vi "RT Driver VI.vi"(6 "Device Clock":string, 9 "Device Inputs FIFO":refnum<k33>, 10 "Device Outputs FIFO":refnum<k33>, 11 "Device Reference":T1 format="%.0x") -> ()   [LabVIEW 2016, in "UDP CD Engine.lvlib"]
uses:
  <vilib>/NI Veristand/Custom Device API/Custom Device Item Ref.ctl
  <vilib>/NI Veristand/Custom Device API/Custom Device Channel Type.ctl
  <vilib>/NI Veristand/Custom Device API/Message Response (String).ctl
  <vilib>/NI Veristand/Custom Device API/Message Response (Byte Array).ctl
  UDP CD Engine.lvlib
  <vilib>/NI Veristand/Custom Device API/Custom Device API.lvlib
  <vilib>/NI Veristand/Custom Device Tools/Custom Device Utility Library/Custom Device Utility Library.lvlib
panel:
  in  "Initialization Status Notifier":refnum<notifier>
  in  "Status Notifier":refnum<notifier>
  # "Custom Device Template\nv1.0"
  # "Use this template as a starting point for creating a custom device code module. The input controls shown here are specially named controls that the system will use to provide the device loop with data. The controls are not required for the device loop to run. For instance, if the device doesn't produce any output data, then you don't need the Device Outputs FIFO control. If you do use these controls, however, they need to have these exact names to be functional."
  # "The optional status notifier element is used to notify the RT engine of the last state of the custom device, and to indicate the device has completed execution. If this control is not used, a default No Error value is returned to the system when the device finishes execution.\n\nNote: This error state is not checked until the system shuts down. Use an output status channel to send more immediate status values to the system."
  # "This optional input can be used to send the VeriStand Engine the final status of the custom device initalization process. If this control exists on the custom device front panel, the VeriStand Engine will wait for a status update before starting up. If the custom device reports an error, that will abort the execution of the current configuration in the VeriStand Engine.\n\nThis control can be deleted if the custom device does not need to send the initialization status update."
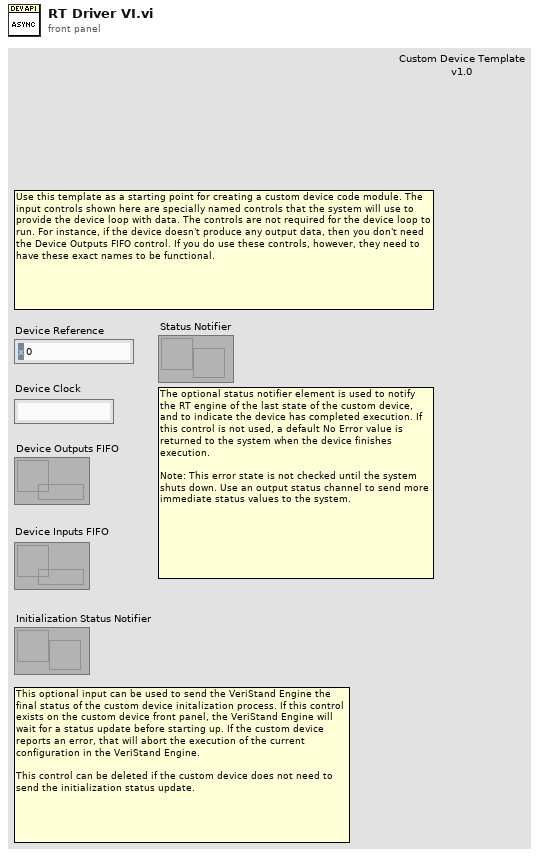
[diagram p1: front panel]
types:
  T1 = typedef "Custom Device API.lvlib/Custom Device Item Ref.ctl" = u64
  T2 = typedef "Custom Device API.lvlib/Custom Device Channel Type.ctl" = enum16{"Input", "Output"}
  T3 = typedef "Custom Device API.lvlib/Custom Device Engine Event Ref.ctl" = refnum<event-registration>
  T4 = typedef "Custom Device API.lvlib/Message Response (String).ctl" = cluster{"Response":string, "Error":errorcluster}
  T5 = typedef "Custom Device API.lvlib/Message Response (Byte Array).ctl" = cluster{"Response":u8[], "Error":errorcluster}
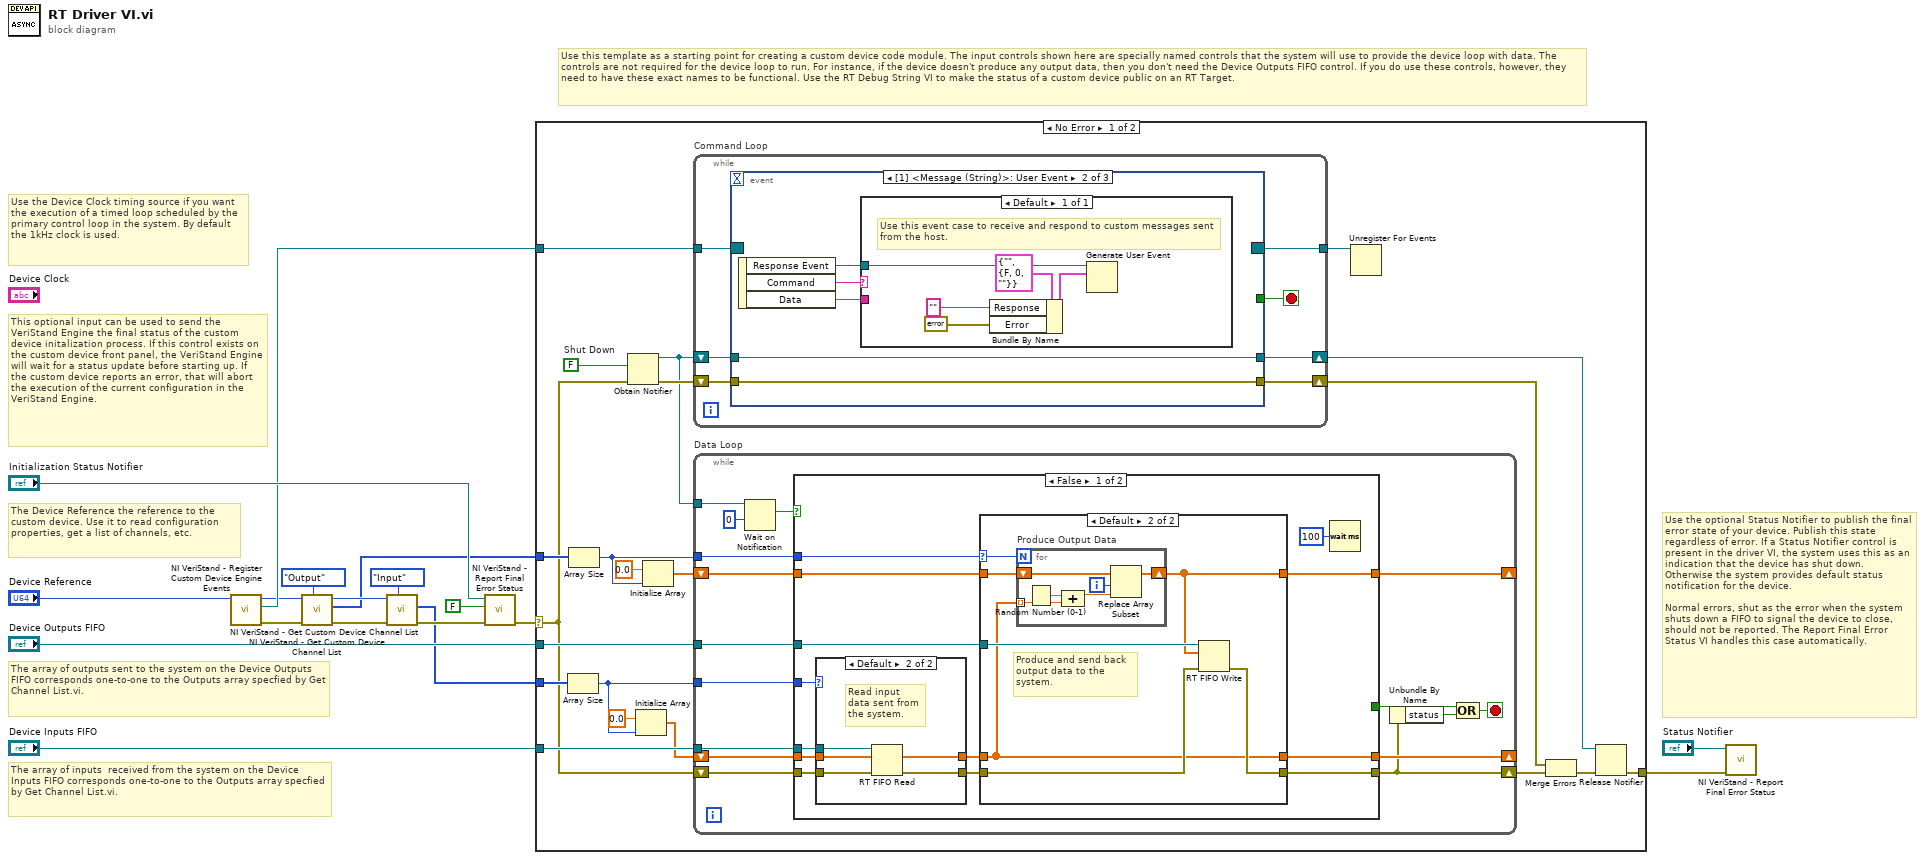
[diagram p0: block diagram]
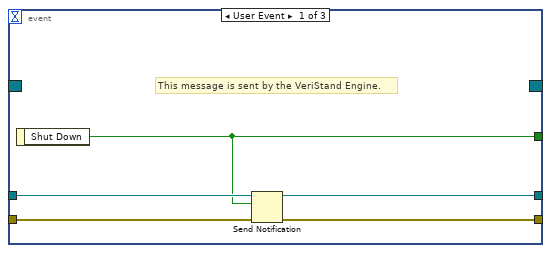
[diagram p2: hidden frame]
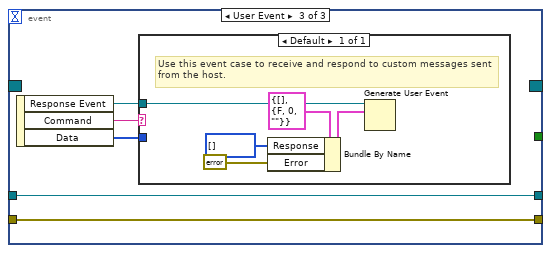
[diagram p3: hidden frame]
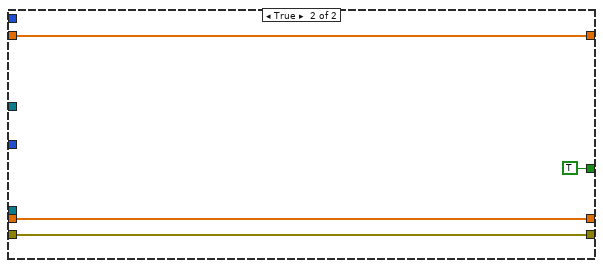
[diagram p6: hidden frame]
diagram:
  # "This optional input can be used to send the VeriStand Engine the final status of the custom device initalization process. If this control exists on the custom device front panel, the VeriStand Engine will wait for a status update before starting up. If the custom device reports an error, that will abort the execution of the current configuration in the VeriStand Engine."
  # "The array of inputs  received from the system on the Device Inputs FIFO corresponds one-to-one to the Outputs array specfied by Get Channel List.vi."
  # "Use the optional Status Notifier to publish the final error state of your device. Publish this state regardless of error. If a Status Notifier control is present in the driver VI, the system uses this as an indication that the device has shut down. Otherwise the system provides default status notification for the device.\n\nNormal errors, shut as the error when the system shuts down a FIFO to signal the device to close, should not be reported. The Report Final Error Status VI handles this case automatically."
  # "The array of outputs sent to the system on the Device Outputs FIFO corresponds one-to-one to the Outputs array specfied by Get Channel List.vi."
  # "The Device Reference the reference to the custom device. Use it to read configuration properties, get a list of channels, etc."
  # "Use the Device Clock timing source if you want the execution of a timed loop scheduled by the primary control loop in the system. By default the 1kHz clock is used."
  # "Use this template as a starting point for creating a custom device code module. The input controls shown here are specially named controls that the system will use to provide the device loop with data. The controls are not required for the device loop to run. For instance, if the device doesn't produce any output data, then you don't need the Device Outputs FIFO control. If you do use these controls, however, they need to have these exact names to be functional. Use the RT Debug String VI to make the status of a custom device public on an RT Target."
  n1 = call <vilib>:"NI VeriStand - Register Custom Device Engine Events.vi"("Device Ref in"="Device Reference") -> ("error out"=w18:errorcluster, "Custom Device Engine Event Ref"=w6:T3, "Device Ref out"=w3:T1)  [unwired: 8 in]
  n2 = call <vilib>:"NI VeriStand - Get Custom Device Channel List.vi"("Channel Type"=Custom_Device_Channel_Type."Output", "error in (no error)"=w18, "Device Ref in"=w3) -> ("error out"=w11:errorcluster, "Specified Channel Ref List"=w8:T1[], "Device Ref out"=w12:T1)  [unwired: 6 out]
  n3 = call <vilib>:"NI VeriStand - Get Custom Device Channel List.vi"("Channel Type"=Custom_Device_Channel_Type."Input", "error in (no error)"=w11, "Device Ref in"=w12) -> ("error out"=w17:errorcluster, "Specified Channel Ref List"=w9:T1[])  [unwired: 7 out]
  n4 = call <vilib>:"NI VeriStand - Report Final Error Status.vi"("error in (no error)"=w17, "Filter FIFO & Shutdown Errors (T)"=FALSE ("Filter FIFO Errors (T)"), "Status Notifier"="Initialization Status Notifier") -> ("error out"=w2:errorcluster)  [unwired: 8 out]
  n5 = case shown="No Error" w2 {
    selector: w2 -> [w21 w128]
    tunnel: "Device Outputs FIFO" -> [w38 _]
    tunnel: "Device Inputs FIFO" -> [w37 _]
    tunnel: w9 -> [w31 _]
    tunnel: w8 -> [w30 _]
    tunnel: w6 -> [w28 _]
    tunnel: [w26 w128] -> w5
    frame No Error {
      w27 = FALSE  # Shut Down
      n6 = Array Size(array=w31) -> (size(s)=w29:i32)
      n7 = Array Size(array=w30) -> (size(s)=w32:i32)
      n8 = Obtain Notifier(notification data type=w27, error in (no error)=w21) -> (notifier out=w24:refnum<notifier>, error out=w39:errorcluster)  [unwired: 2 in, 1 out]
      n9 = Initialize Array(0.0 ("element"), w29) -> (w33:dbl[])
      n10 = Initialize Array(0.0 ("element"), w32) -> (w34:dbl[])
      n11 = while "Command Loop" {
        tunnel: w28 -> [w46]
        tunnel: [w45] -> w25
        shift-right: [w42] -> w23
        shift-left: w24 -> [w43]
        shift-right: [w40] -> w19
        shift-left: w39 -> [w41]
        stop <- w44 stop-if-true
        n12 = event shown="[1] <Message (String)>: User Event" {
          selector: w46 -> [_ _ _]
          dyn-events: [_ _ _] -> w45
          timeout: _ -> [_ _ _]
          tunnel: [w49 _ _] -> w44
          tunnel: w43 -> [w50 w54 w64]
          tunnel: [w51 w54 w64] -> w42
          tunnel: w41 -> [w48 w52 w62]
          tunnel: [w47 w52 w62] -> w40
          event User Event {
            # "This message is sent by the VeriStand Engine."
            n13 = event-data() -> ("Shut Down"=w49:bool)  [unwired: 1 in]
            n14 = Send Notification(notification=w49, notifier=w50, error in (no error)=w48) -> (notifier out=w51:refnum<notifier>, error out=w47:errorcluster)
          }
          event User Event {
            n15 = event-data() -> ("Response Event"=w53:refnum<user-event>, "Command"=w56:string, "Data"=w55:string)  [unwired: 1 in]
            n16 = case shown="Default" w56 {
              tunnel: w55 -> [_]
              tunnel: w53 -> [w61]
              frame Default {
                # "Use this event case to receive and respond to custom messages sent from the host."
                n17 = Bundle By Name(cluster=T4 {"Response"="", "Error"={"status"=FALSE, "code"=0, "source"=""}} ("event data"), "Response"="", "Error"=errorcluster {"status"=FALSE, "code"=0, "source"=""}) -> (w59:T4)
                n18 = Generate User Event(user event=w61, event data cluster=w59) -> ()  [unwired: 2 in, 2 out]
              }
            }
          }
          event User Event {
            n19 = event-data() -> ("Response Event"=w63:refnum<user-event>, "Command"=w66:string, "Data"=w65:u8[])  [unwired: 1 in]
            n20 = case shown="Default" w66 {
              tunnel: w65 -> [_]
              tunnel: w63 -> [w71]
              frame Default {
                # "Use this event case to receive and respond to custom messages sent from the host."
                n21 = Bundle By Name(cluster=T5 {"Response"=[], "Error"={"status"=FALSE, "code"=0, "source"=""}} ("event data"), "Response"=u8[] [], "Error"=errorcluster {"status"=FALSE, "code"=0, "source"=""}) -> (w68:T5)
                n22 = Generate User Event(user event=w71, event data cluster=w68) -> ()  [unwired: 2 in, 2 out]
              }
            }
          }
        }
      }
      n23 = while "Data Loop" {
        shift-right: [w85] -> _
        shift-left: w33 -> [w86]
        shift-right: [w77] -> w22
        shift-left: w21 -> [w87]
        shift-right: [w83] -> _
        shift-left: w34 -> [w84]
        tunnel: w32 -> [w80]
        tunnel: w38 -> [w82]
        tunnel: w37 -> [w81]
        tunnel: w29 -> [w79]
        tunnel: w24 -> [w76]
        stop <- w72 stop-if-true
        n24 = Wait on Notification(notifier=w76, timeout in ms (-1)=0) -> (notification=w75:bool)  [unwired: 2 in, 3 out]
        n25 = case shown="False" w75 {
          tunnel: w87 -> [w100 w126]
          tunnel: w86 -> [w99 w127]
          tunnel: [w98 w127] -> w85
          tunnel: w84 -> [w97 w125]
          tunnel: [w96 w125] -> w83
          tunnel: w82 -> [w95 _]
          tunnel: w81 -> [w94 _]
          tunnel: w80 -> [w93 _]
          tunnel: w79 -> [w92 _]
          tunnel: [w89 w126] -> w77
          tunnel: [_ TRUE] -> w73
          frame False {
            n26 = case shown="Default" w92 {
              tunnel: w94 -> [_ w123]
              tunnel: w99 -> [w118 w122]
              tunnel: [w118 w121] -> w91
              tunnel: [w117 w120] -> w90
              tunnel: w100 -> [w117 w119]
              frame 0 {
                # "No inputs to read\nfrom system. Inputs FIFO not created in this case, so don't write to it."
              }
              frame Default {
                # "Read input data sent from the system."
                n27 = RT FIFO Read(0:w123, 1:w122, 3:w119) -> (9:w121:dbl[], 11:w120:errorcluster)  [unwired: 4 out]
              }
            }
            n28 = case shown="Default" w93 {
              selector: w93 -> [_ w104]
              tunnel: w95 -> [_ w110]
              tunnel: w97 -> [w103 w109]
              tunnel: w91 -> [w102 w105]
              tunnel: w90 -> [w101 w108]
              tunnel: [w101 w107] -> w89
              tunnel: [w103 w106] -> w96
              tunnel: [w102 w105] -> w98
              frame 0 {
                # "No outputs to write to system. The Device Outputs FIFO is never created in this case, so don't write to it."
              }
              frame Default {
                # "Produce and send back output data to the system."
                n29 = for "Produce Output Data" {
                  N: w104 -> [_]
                  shift-right: [w115] -> w106
                  shift-left: w109 -> [w116]
                  tunnel: w105 -> [w111] mode=indexing
                  i -> [w114]
                  n30 = Random Number (0-1)() -> (number: 0 to 1=w113:dbl)
                  n31 = Compound Arithmetic op=ADD(w113, w111) -> (w112:dbl)
                  n32 = Replace Array Subset(array=w116, new element=w112, index=w114) -> (w115:dbl[])
                }
                n33 = RT FIFO Write(0:w110, 1:w106, 3:w108) -> (11:w107:errorcluster)  [unwired: 1 in, 4 out]
              }
            }
            n34 = Wait (ms)(milliseconds to wait=u32 100) -> ()  [unwired: 1 out]
          }
          frame True {
          }
        }
        n35 = Unbundle By Name(w77) -> ("status"=w74:bool)
        n36 = Compound Arithmetic op=OR(w73, w74) -> (w72:bool)
      }
      n37 = Unregister For Events(event registration refnum=w25) -> ()  [unwired: 1 in, 1 out]
      n38 = Merge Errors(w19, w22) -> (w20:errorcluster)
      n39 = Release Notifier(notifier=w23, error in (no error)=w20) -> (error out=w26:errorcluster)  [unwired: 1 in, 2 out]
    }
    frame Error {
    }
  }
  n40 = call <vilib>:"NI VeriStand - Report Final Error Status.vi"("error in (no error)"=w5, "Status Notifier"="Status Notifier") -> ()  [unwired: 1 in, 9 out]
